vi "Set Motor Outputs.vi"(11 "Updated Drive Metrics in":T1) -> (3 "Updated Drive Metrics out":T1)   [LabVIEW 2013]
uses:
  Drive Train Metrics.ctl
  CmdFlag.ctl
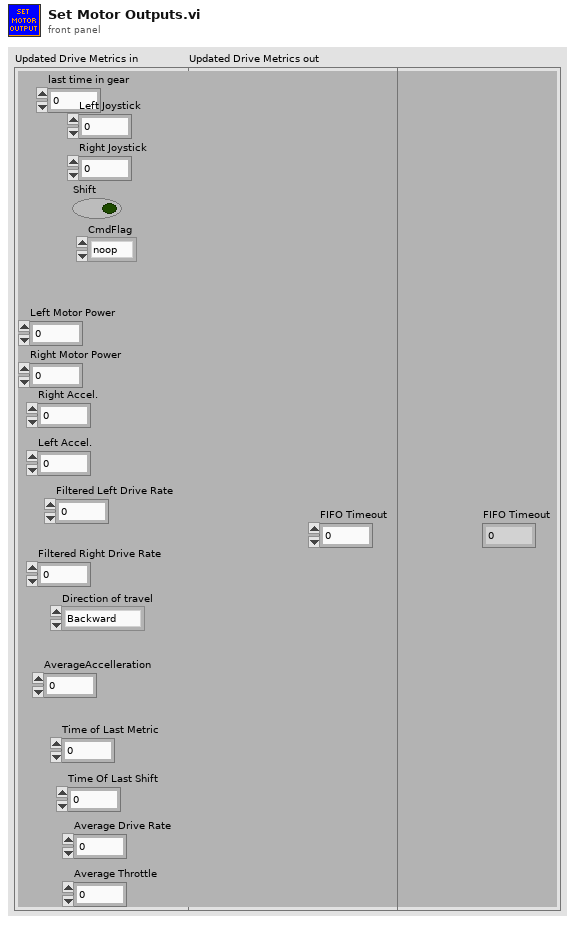
[diagram p1: front panel]
types:
  T1 = typedef "Drive Train Metrics.ctl" = cluster{"last time in gear":u32, "Shift":bool, "Right Joystick":dbl, "Left Joystick":dbl, "CmdFlag":T2, "Right Motor Power":dbl, "Left Motor Power":dbl, "Right Accel.":dbl, "Left Accel.":dbl, "Filtered Left Drive Rate":dbl, "Filtered Right Drive Rate":dbl, "Direction of travel":enum16{"Backward", "Forward", "Spin"}, "AverageAccelleration":dbl, "Time of Last Metric":u32, "Time Of Last Shift":dbl, "Average Drive Rate":dbl, "Average Throttle":dbl, "FIFO Timeout":i32}
  T2 = typedef "CmdFlag.ctl" = enum16{"noop", "suspend", "resume"}
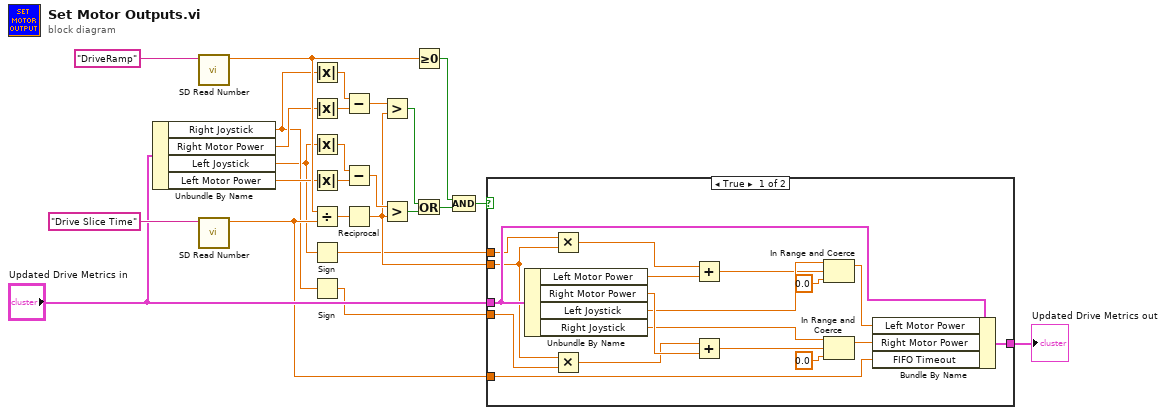
[diagram p0: block diagram]
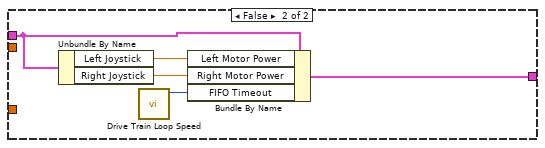
[diagram p2: hidden frame]
diagram:
  n1 = Unbundle By Name("Updated Drive Metrics in") -> ("Right Joystick"=w5:dbl, "Right Motor Power"=w16:dbl, "Left Joystick"=w3:dbl, "Left Motor Power"=w19:dbl)
  n2 = call <vilib>:"SD Read Number.vi"("Name"="DriveRamp") -> ("Numeric"=w20:dbl)  [unwired: 8 in, 2 out]
  n3 = call <vilib>:"SD Read Number.vi"("Name"="Drive Slice Time") -> ("Numeric"=w11:dbl)  [unwired: 8 in, 2 out]
  n4 = Absolute Value(x=w5) -> (abs(x)=w17:dbl)
  n5 = Absolute Value(x=w16) -> (abs(x)=w15:dbl)
  n6 = Absolute Value(x=w3) -> (abs(x)=w4:dbl)
  n7 = Absolute Value(x=w19) -> (abs(x)=w18:dbl)
  n8 = Divide(x=w20, y=w11) -> (x/y=w10:dbl)
  n9 = Sign(1:w3) -> (0:w1:dbl)
  n10 = Sign(1:w5) -> (0:w2:dbl)
  n11 = Subtract(x=w17, y=w15) -> (x-y=w23:dbl)
  n12 = Subtract(x=w4, y=w18) -> (x-y=w22:dbl)
  n13 = Reciprocal(x=w10) -> (1/x=w9:dbl)
  n14 = Greater?(x=w23, y=w9) -> (0:w6:bool)
  n15 = Greater?(x=w22, y=w9) -> (0:w7:bool)
  n16 = Greater Or Equal To 0?(x=w20) -> (x >= 0?=w24:bool)
  n17 = Or(x=w6, y=w7) -> (x .or. y?=w8:bool)
  n18 = Compound Arithmetic op=AND(w24, w8) -> (w14:bool)
  n19 = case shown="True" w14 {
    tunnel: "Updated Drive Metrics in" -> [w43 w46]
    tunnel: [w42 w45] -> w12
    tunnel: w11 -> [w41 _]
    tunnel: w9 -> [w35 _]
    tunnel: w2 -> [w38 _]
    tunnel: w1 -> [w36 _]
    frame True {
      n20 = Unbundle By Name(w43) -> ("Left Motor Power"=w40:dbl, "Right Motor Power"=w39:dbl, "Left Joystick"=w32:dbl, "Right Joystick"=w27:dbl)
      n21 = Multiply(x=w36, y=w35) -> (x*y=w34:dbl)
      n22 = Multiply(x=w35, y=w38) -> (x*y=w37:dbl)
      n23 = Add(x=w34, y=w40) -> (x+y=w31:dbl)
      n24 = Add(x=w37, y=w39) -> (x+y=w28:dbl)
      n25 = In Range and Coerce(upper limit=w32, x=w31, lower limit=0.0) -> (coerced(x)=w30:dbl)  [unwired: 1 out]
      n26 = In Range and Coerce(upper limit=w27, x=w28, lower limit=0.0) -> (coerced(x)=w26:dbl)  [unwired: 1 out]
      n27 = Bundle By Name(cluster=w43, "Left Motor Power"=w30, "Right Motor Power"=w26, "FIFO Timeout"=w41) -> (w42:T1)
    }
    frame False {
      n28 = Unbundle By Name(w46) -> ("Left Joystick"=w47:dbl, "Right Joystick"=w48:dbl)
      n29 = call "Drive Train Loop Speed.vi"() -> ("FIFO Timeout"=w44:i32)  [unwired: 11 in]
      n30 = Bundle By Name(cluster=w46, "Left Motor Power"=w47, "Right Motor Power"=w48, "FIFO Timeout"=w44) -> (w45:T1)
    }
  }
  "Updated Drive Metrics out" <- w12
